vi "UHR-Fleezers Control (host) - 12.1.vi"() -> ()   [LabVIEW 2012] (continued)
          tunnel: "Setpoints (V)" -> [w3405 w3420]
          tunnel: w3394 -> [_ w3414]
          frame False {
            n2043 = Multiply(x=3276.7, y=w3405) -> (x*y=w3406:cluster{"Set 1":dbl, "Set 2":dbl})
            n2044 = To Word Integer(number=w3406) -> (16bit integer=w3404:cluster{"Set 1":i16, "Set 2":i16})
          }
          frame True {
            n2045 = Unbundle By Name(w3414) -> ("Set 1"=w3413:dbl, "Set 2"=w3412:dbl)
            n2046 = Unbundle By Name(w3420) -> ("Set 1"=w3419:dbl, "Set 2"=w3418:dbl)
            n2047 = Unbundle By Name(w3417) -> ("Set 1"=w3416:bool, "Set 2"=w3415:bool)
            n2048 = Select(t=w3413, s=w3416, f=w3419) -> (s? t:f=w3411:dbl)
            n2049 = Select(t=w3412, s=w3415, f=w3418) -> (s? t:f=w3410:dbl)
            n2050 = Bundle By Name(cluster=w3420, "Set 1"=w3411, "Set 2"=w3410) -> (w3408:cluster{"Set 1":dbl, "Set 2":dbl})
            n2051 = local write "Setpoints (V)"(w3408) -> ()
            n2052 = Multiply(x=3276.7, y=w3408) -> (x*y=w3409:cluster{"Set 1":dbl, "Set 2":dbl})
            n2053 = To Word Integer(number=w3409) -> (16bit integer=w3421:cluster{"Set 1":i16, "Set 2":i16})
          }
        }
        n2054 = Unbundle By Name(w3393) -> ("Set 1"=w3392:i16, "Set 2"=w3391:i16)
        n2055 = xnode "Read/Write Control"("FPGA VI Reference In"=w3389, "error in"=w3388, "FB Setpoint Set 1"=w3392, "FB Setpoint Set 2"=w3391) -> ("error out"=w3387:errorcluster)  [unwired: 1 out]
      }
      event "Invert GI": Value Change {
        n2056 = event-data() -> ()  [unwired: 7 out]
        n2057 = xnode "Read/Write Control"("FPGA VI Reference In"=w3426, "error in"=w3424, "Invert GI"="Invert GI", "Invert GI 2"="Invert GI") -> ("error out"=w3425:errorcluster)  [unwired: 1 out]
      }
      event "Green FB Setpoint (mV)", "Green FB Gains", "Green FB On/Off", "Current When FB OFF (%)", "Green int current ON count adj": Value Change {
        n2058 = event-data() -> ()  [unwired: 7 out]
        n2059 = local read "Green FB Setpoint (mV)"() -> (w3437:dbl)
        n2060 = local read "Current When FB OFF (%)"() -> (w3440:dbl)
        n2061 = Multiply(x=w3437, y=3.2767) -> (x*y=w3436:dbl)
        n2062 = Multiply(x=w3440, y=655.35) -> (x*y=w3441:dbl)
        n2063 = To Unsigned Word Integer(number=w3441) -> (unsigned 16bit integer=w3439:u16)
        n2064 = local read "Green int current ON count adj"() -> (w3443:u32)
        n2065 = local read "Green Laser ON/Interlacing"() -> (w3434:bool)
        n2066 = local read "Green FB Gains"() -> (w3430:T9)
        n2067 = local read "Green laser mode"() -> (w3433:enum32{"Laser ON", "Laser OFF", "Interlace"})
        n2068 = local read "Green FB On/Off"() -> (w3444:bool)
        n2069 = Equal?(x=w3433, y=enum32{"Laser ON", "Laser OFF", "Interlace"}."Interlace") -> (x = y?=w3431:bool)
        n2070 = Unbundle By Name(w3430) -> ("proportional gain (Kc)"=w3429:i16, "integral gain (Kc*Ts/Ti)"=w3428:i16, "derivative gain (Kc*Td/Ts)"=w3427:i16)
        n2071 = Compound Arithmetic op=AND(w3431, w3444, w3434) -> (w3435:bool)
        n2072 = xnode "Read/Write Control"("FPGA VI Reference In"=w3447, "error in"=w3446, "Green FB Setpoint"=w3436, "Green FB On/Off"=w3435, "Current Out"=w3439, "Green int current ON count adj"=w3443, "P3"=w3429, "I3"=w3428, "D3"=w3427) -> ("error out"=w3445:errorcluster)  [unwired: 1 out]
      }
      event "Green laser mode", "Green Laser ON/Interlacing": Value Change {
        n2073 = event-data() -> ()  [unwired: 7 out]
        n2074 = local write "Green Laser ON/OFF"("Green Laser ON/Interlacing") -> ()
        n2075 = case shown="True" "Green Laser ON/Interlacing" {
          tunnel: "Green laser mode" -> [_ w3461]
          tunnel: [enum32{"Laser ON", "Laser OFF", "Interlace"}."Laser OFF" ("Green laser mode") w3461] -> w3450
          tunnel: [FALSE w3457] -> w3449
          frame False {
          }
          frame True {
            n2076 = local read "Green FB On/Off"() -> (w3458:bool)
            n2077 = Equal?(x=w3461, y=enum32{"Laser ON", "Laser OFF", "Interlace"}."Interlace") -> (x = y?=w3459:bool)
            n2078 = And(x=w3459, y=w3458) -> (x .and. y?=w3457:bool)
          }
        }
        n2079 = xnode "Read/Write Control"("FPGA VI Reference In"=w3454, "error in"=w3452, "Operating Mode"=w3450, "Operating Mode 2"=w3450, "Green FB On/Off"=w3449) -> ("error out"=w3453:errorcluster)  [unwired: 1 out]
      }
      event "Green Laser ON/OFF": Value Change {
        n2080 = event-data() -> ()  [unwired: 7 out]
        n2081 = property on="Green Laser ON/Interlacing" class="Bool (strict)"("Val(Sgnl)"="Green Laser ON/OFF") -> ()  [unwired: 2 in, 2 out]
      }
      event "Test ttrig": Value Change {
        n2082 = event-data() -> ()  [unwired: 7 out]
        n2083 = xnode "Read/Write Control"("FPGA VI Reference In"=w3466, "error in"=w3465, "TTrig?"=TRUE) -> ("error out"=w3464:errorcluster)  [unwired: 1 out]
      }
      event "Neg. TTrig FPGA": Value Change {
        n2084 = event-data() -> ()  [unwired: 7 out]
        n2085 = xnode "Read/Write Control"("FPGA VI Reference In"=w3470, "error in"=w3469, "TTrig Negate Pos"="Neg. TTrig FPGA") -> ()  [unwired: 2 out]
      }
      event "- phase (APD 1 Gate)", "+ phase (APD 1 Gate)": Value Change {
        n2086 = event-data() -> ()  [unwired: 7 out]
        n2087 = local read "Phase Adj. (APD 1 Gate)"() -> (w3471:i16)
        n2088 = Negate(x=w3471) -> (-x=w3479:i16)
        n2089 = Select(t=w3479, s="- phase (APD 1 Gate)", f=w3471) -> (s? t:f=w3478:i16)
        n2090 = Or(x="- phase (APD 1 Gate)", y="+ phase (APD 1 Gate)") -> (x .or. y?=w3474:bool)
        n2091 = xnode "Read/Write Control"("FPGA VI Reference In"=w3481, "error in"=w3480, "Phase count adjustment (APD 1 Gate)"=w3478) -> ("FPGA VI Reference Out"=w3476:T18, "error out"=w3477:errorcluster)
        n2092 = xnode "Read/Write Control"("FPGA VI Reference In"=w3476, "error in"=w3477, "+ phase (APD 1 Gate)"=w3474) -> ("error out"=w3475:errorcluster)  [unwired: 1 out]
      }
      event "+ phase (APD 2 Gate)", "- phase (APD 2 Gate)": Value Change {
        n2093 = event-data() -> ()  [unwired: 7 out]
        n2094 = local read "Phase Adj. (APD 2 Gate)"() -> (w3482:i16)
        n2095 = Negate(x=w3482) -> (-x=w3490:i16)
        n2096 = Select(t=w3490, s="- phase (APD 2 Gate)", f=w3482) -> (s? t:f=w3489:i16)
        n2097 = Or(x="- phase (APD 2 Gate)", y="+ phase (APD 2 Gate)") -> (x .or. y?=w3485:bool)
        n2098 = xnode "Read/Write Control"("FPGA VI Reference In"=w3492, "error in"=w3491, "Phase count adjustment (APD 2 Gate)"=w3489) -> ("FPGA VI Reference Out"=w3487:T18, "error out"=w3488:errorcluster)
        n2099 = xnode "Read/Write Control"("FPGA VI Reference In"=w3487, "error in"=w3488, "+ phase (APD 2 Gate)"=w3485) -> ("error out"=w3486:errorcluster)  [unwired: 1 out]
      }
      event "Phase Adj. (APD Acq)", "+ phase (APD Acq)", "- phase (APD Acq)": Value Change {
        n2100 = event-data() -> ()  [unwired: 7 out]
        n2101 = local read "Phase Adj. (APD Acq)"() -> (w3495:i16)
        n2102 = Negate(x=w3495) -> (-x=w3501:i16)
        n2103 = Select(t=w3501, s="+ phase (APD Acq)", f=w3495) -> (s? t:f=w3500:i16)
        n2104 = Or(x="+ phase (APD Acq)", y="- phase (APD Acq)") -> (x .or. y?=w3496:bool)
        n2105 = xnode "Read/Write Control"("FPGA VI Reference In"=w3503, "error in"=w3502, "Phase Count Adjustment (APD Acq)"=w3500) -> ("FPGA VI Reference Out"=w3498:T18, "error out"=w3499:errorcluster)
        n2106 = xnode "Read/Write Control"("FPGA VI Reference In"=w3498, "error in"=w3499, "+ phase (APD Acq)"=w3496) -> ("error out"=w3497:errorcluster)  [unwired: 1 out]
      }
      event "Phase adj. (GI)", "+ phase (GI)", "- phase (GI)": Value Change {
        n2107 = event-data() -> ()  [unwired: 7 out]
        n2108 = Negate(x="Phase adj. (GI)") -> (-x=w3512:i16)
        n2109 = Select(t=w3512, s="+ phase (GI)", f="Phase adj. (GI)") -> (s? t:f=w3511:i16)
        n2110 = Or(x="+ phase (GI)", y="- phase (GI)") -> (x .or. y?=w3507:bool)
        n2111 = xnode "Read/Write Control"("FPGA VI Reference In"=w3514, "error in"=w3513, "Phase count adjustment (GI)"=w3511) -> ("FPGA VI Reference Out"=w3509:T18, "error out"=w3510:errorcluster)
        n2112 = xnode "Read/Write Control"("FPGA VI Reference In"=w3509, "error in"=w3510, "+ phase (GI)"=w3507) -> ("error out"=w3508:errorcluster)  [unwired: 1 out]
      }
      event "Phase adj. (GI) 2", "+ phase (GI) 2", "- phase (GI) 2": Value Change {
        n2113 = event-data() -> ()  [unwired: 7 out]
        n2114 = Negate(x="Phase adj. (GI) 2") -> (-x=w3523:i16)
        n2115 = Select(t=w3523, s="+ phase (GI) 2", f="Phase adj. (GI) 2") -> (s? t:f=w3522:i16)
        n2116 = Or(x="+ phase (GI) 2", y="- phase (GI) 2") -> (x .or. y?=w3518:bool)
        n2117 = xnode "Read/Write Control"("FPGA VI Reference In"=w3525, "error in"=w3524, "Phase count adjustment (GI) 2"=w3522) -> ("FPGA VI Reference Out"=w3520:T18, "error out"=w3521:errorcluster)
        n2118 = xnode "Read/Write Control"("FPGA VI Reference In"=w3520, "error in"=w3521, "+ phase (GI) 2"=w3518) -> ("error out"=w3519:errorcluster)  [unwired: 1 out]
      }
      event "Phase adj. (Green FB)", "- phase (Green FB)", "+ phase (Green FB)": Value Change {
        n2119 = event-data() -> ()  [unwired: 7 out]
        n2120 = Negate(x="Phase adj. (Green FB)") -> (-x=w3534:i16)
        n2121 = Select(t=w3534, s="+ phase (Green FB)", f="Phase adj. (Green FB)") -> (s? t:f=w3533:i16)
        n2122 = Or(x="+ phase (Green FB)", y="- phase (Green FB)") -> (x .or. y?=w3529:bool)
        n2123 = xnode "Read/Write Control"("FPGA VI Reference In"=w3536, "error in"=w3535, "Phase count adjustment (Green FB)"=w3533) -> ("FPGA VI Reference Out"=w3531:T18, "error out"=w3532:errorcluster)
        n2124 = xnode "Read/Write Control"("FPGA VI Reference In"=w3531, "error in"=w3532, "+ phase (Green FB)"=w3529) -> ("error out"=w3530:errorcluster)  [unwired: 1 out]
      }
      event "Invert APD Gate", "APD Gate ON Count", "APD Gate OFF Count", "APD Gate", "APD Integration Time (s)", "APD 1 AO Mult.", "APD 2 AO Mult.", "On one out of X cycles": Value Change {
        n2125 = event-data() -> ()  [unwired: 7 out]
        n2126 = Add(x="GI Frequency, ON count", y="GI Frequency, OFF count") -> (x+y=w3540:u32)
        n2127 = Add(x="APD Gate ON Count", y="APD Gate OFF Count") -> (x+y=w3553:u32)
        n2128 = Multiply(x="On one out of X cycles", y=w3540) -> (x*y=w3537:u32)
        "Green FB Count" <- w3537
        n2129 = Subtract(x=w3537, y="GI Frequency, ON count") -> (x-y=w3538:u32)
        n2130 = Multiply(x=w3553, y="On one out of X cycles") -> (x*y=w3552:u32)
        n2131 = Subtract(x=w3552, y="APD Gate ON Count") -> (x-y=w3551:u32)
        n2132 = local read "DMA Update Period (s)"() -> (w3554:dbl)
        n2133 = Multiply(x="APD Integration Time (s)", y=40000000.0) -> (x*y=w3559:dbl)
        n2134 = Reciprocal(x="APD Integration Time (s)") -> (1/x=→"APD Acq Rate (Hz)":dbl)
        n2135 = To Unsigned Long Integer(number=w3559) -> (unsigned 32bit integer=w3543:u32)
        "APD Int. Count" <- w3543
        n2136 = xnode "Read/Write Control"("FPGA VI Reference In"=w3563, "error in"=w3562, "Invert APD Gate"="Invert APD Gate", "APD Gate ON Count"="APD Gate ON Count", "APD Gate OFF Count"=w3551, "APD Acq Rate Count"=w3543, "APD Gate Operating Mode"="APD Gate", "APD 1 AO scale factor"="APD 1 AO Mult.", "APD 2 AO scale factor"="APD 2 AO Mult.", "Green interlace ON count"="GI Frequency, ON count", "Green interlace OFF count"=w3538, "Green interlace ON count 2"="GI Frequency, ON count", "Green interlace OFF count 2"=w3538, "Green FB Count"=w3537) -> ("error out"=w3561:errorcluster)  [unwired: 1 out]
        n2137 = Divide(x=w3554, y="APD Integration Time (s)") -> (x/y=w3557:dbl)
        n2138 = Multiply(x=2.0, y=w3557) -> (x*y=w3556:dbl)
        n2139 = local write "APD Samples/FIFO Acq."(w3557) -> ()
        n2140 = local write "APD Elements/DMA read"(w3556) -> ()
      }
      event "Number of F/B Scans (AOD)", "Scan Speed (nm/s)", "Scan BD", "Initial delta (MHz)", "Step Size (nm)", "Scan Range (nm)": Value Change {
        w3625 = 123.0  # AOM cal (nm/MHz)
        n2141 = event-data() -> ()  [unwired: 7 out]
        n2142 = local read "BD 1 Frequency 1 (MHz)"() -> (w3608:dbl)
        n2143 = local read "AOM X Cal (nm/MHz)"() -> (w3600:dbl)
        n2144 = local read "X RF Frequency Limits (MHz)"() -> (w3612:T15)
        n2145 = local read "Y RF Frequency Limits (MHz)"() -> (w3609:T15)
        n2146 = local read "BD 2 Frequency 1 (MHz)"() -> (w3614:dbl)
        n2147 = Negate(x="Scan Range (nm)") -> (-x=w3578:dbl)
        n2148 = Divide(x=w3578, y=w3600) -> (x/y=w3582:dbl)
        n2149 = Select(t=w3612, s="Scan BD", f=w3609) -> (s? t:f=w3611:T15)
        n2150 = Select(t=w3608, s="Scan BD", f=w3614) -> (s? t:f=w3613:dbl)
        n2151 = Unbundle By Name(w3611) -> ("Maximum"=w3620:dbl, "Minimum"=w3619:dbl)
        n2152 = Add(x=w3582, y=w3613) -> (x+y=w3617:dbl)
        n2153 = Divide(x=w3578, y="Step Size (nm)") -> (x/y=w3597:dbl)
        n2154 = Divide(x="Step Size (nm)", y=w3600) -> (x/y=w3606:dbl)
        n2155 = Absolute Value(x=w3597) -> (abs(x)=w3581:dbl)
        n2156 = Sign(1:w3578) -> (0:w3579:dbl)
        n2157 = In Range and Coerce(upper limit=w3620, x=w3617, lower limit=w3619) -> (coerced(x)=w3616:dbl, In Range?=w3618:bool)
        n2158 = To Unsigned Quad Integer(1:w3581) -> (0:w3596:u64)
        "Scan steps (AOD)" <- w3596
        n2159 = call "IR AOM freq to word.vi"("Frequency In (MHz)"=w3606) -> ("Frequency Word Out (double)"=w3603:dbl)
        n2160 = Multiply(x=w3579, y=w3603) -> (x*y=w3580:dbl)
        n2161 = Subtract(x=w3617, y=w3616) -> (x-y=w3615:dbl)
        n2162 = To Quad Integer(1:w3580) -> (0:w3602:i64)
        "Incr. int (AOD)" <- w3602
        n2163 = Subtract(x=w3582, y=w3615) -> (x-y=w3601:dbl)
        "Scan Range (MHz)" <- w3601
        n2164 = Select(t=w3582, s=w3618, f=w3601) -> (s? t:f=w3621:dbl)
        n2165 = Multiply(x=w3601, y=w3600) -> (x*y=w3599:dbl)
        n2166 = Decrement(x=w3596) -> (x-1=w3649:u64)
        n2167 = Negate(x=w3599) -> (-x=w3595:dbl)
        n2168 = local write "Scan Range (nm)"(w3595) -> ()
        n2169 = Divide(x=w3621, y=w3649) -> (x/y=w3605:dbl)
        "Scan Increment (MHz)" <- w3605
        n2170 = call "IR AOM freq to word.vi"("Frequency In (MHz)"=w3605) -> ("Frequency Word Out (double)"=w3604:dbl)
        n2171 = Divide(x="Step Size (nm)", y="Scan Speed (nm/s)") -> (x/y=w3592:dbl)
        n2172 = To Quad Integer(1:w3604) -> ()  [unwired: 1 out]
        n2173 = local read "Number Interlace Sets"() -> (w3576:u8)
        n2174 = local read "AI Count (ticks)"() -> (w3577:u32)
        n2175 = local read "Total Counts (ticks)"() -> (w3575:u32)
        n2176 = local read "# Samples/trap"() -> (w3607:u32)
        n2177 = Multiply(x=w3577, y=w3576) -> (x*y=w3574:u32)
        n2178 = Divide(x=w3575, y=w3574) -> (x/y=w3573:dbl)
        n2179 = Select(t=w3608, s="Scan BD", f=w3614) -> (s? t:f=w3646:dbl)
        "Initial freq. (MHz)" <- w3646
        n2180 = Add(x=w3621, y=w3646) -> (x+y=→"Final freq. (MHz)":dbl)
        n2181 = Divide(x=w3575, y=40000000.0) -> (x/y=w3591:dbl)
        n2182 = Divide(x=w3592, y=w3591) -> (x/y=w3590:dbl)
        n2183 = To Unsigned Quad Integer(1:w3590) -> (0:w3565:u64)
        n2184 = Quotient & Remainder(x=w3565, y=u64 2) -> (x-y*floor(x/y)=w3569:u64)  [unwired: 1 out]
        n2185 = Equal?(x=w3569, y=u64 0) -> (x = y?=w3567:bool)
        n2186 = Decrement(x=w3565) -> (x-1=w3566:u64)
        n2187 = Select(t=w3565, s=w3567, f=w3566) -> (s? t:f=w3564:u64)
        "Cycles/step (AOD)" <- w3564
        n2188 = xnode "Read/Write Control"("FPGA VI Reference In"=w3657, "error in"=w3656, "Scan steps"=w3596, "Number of scans"="Number of F/B Scans (AOD)", "Cycles per step"=w3564, "Scan freq.  increment"=w3602, "Scan BD"="Scan BD") -> ("error out"=w3655:errorcluster)  [unwired: 1 out]
        n2189 = Multiply(x=w3596, y=w3564) -> (x*y=w3650:u64)
        n2190 = Multiply(x=w3650, y=u64 2) -> (x*y=w3572:u64)
        n2191 = Multiply(x=w3573, y=w3572) -> (x*y=w3571:dbl)
        "Data points/scan (f/b)" <- w3571
        n2192 = Multiply(x=w3571, y="Number of F/B Scans (AOD)") -> (x*y=w3653:dbl)
        "Data points/scans" <- w3653
        n2193 = Divide(x=w3653, y=w3607) -> (x/y=→"N sets should be saved":dbl)
        n2194 = Multiply(x=w3650, y=w3591) -> (x*y=w3589:dbl)
        "Time/Scan (s) (AOD)" <- w3589
        n2195 = Select(t=w3621, s="Scan BD", f=0.0) -> (s? t:f=w3647:dbl)
        n2196 = Select(t=0.0, s="Scan BD", f=w3621) -> (s? t:f=w3643:dbl)
        n2197 = local read "BD 2 Frequency 2 (MHz)"() -> (w3639:dbl)
        n2198 = local read "BD 1 Frequency 2 (MHz)"() -> (w3642:dbl)
        n2199 = Add(x=w3643, y=w3614) -> (x+y=w3640:dbl)
        n2200 = Add(x=w3608, y=w3647) -> (x+y=w3641:dbl)
        n2201 = Multiply(x=w3589, y=2.0) -> (x*y=w3588:dbl)
        n2202 = Multiply(x=w3588, y="Number of F/B Scans (AOD)") -> (x*y=w3585:dbl)
        n2203 = Divide(x=w3585, y=60.0) -> (x/y=→"Time to Finish All (min)":dbl)
        n2204 = Add(x="Trap 2 Bead Size (nm)", y="Trap 1 Bead Size (nm)") -> (x+y=w3629:dbl)
        n2205 = Divide(x=w3629, y=2.0) -> (x/y=w3623:dbl)
        n2206 = local read "Initial delta (MHz)"() -> (w3626:dbl)
        n2207 = Subtract(x=w3640, y=w3639) -> (x-y=w3637:dbl)
        n2208 = Subtract(x=w3641, y=w3642) -> (x-y=w3638:dbl)
        n2209 = Square(x=w3637) -> (x^2=w3636:dbl)
        n2210 = Square(x=w3638) -> (x^2=w3635:dbl)
        n2211 = Add(x=w3635, y=w3636) -> (x+y=w3634:dbl)
        n2212 = Square Root(x=w3634) -> (sqrt(x)=w3633:dbl)
        "Final delta (MHz)" <- w3633
        n2213 = Multiply(x=w3625, y=w3633) -> (x*y=w3632:dbl)
        n2214 = Multiply(x=w3626, y=w3625) -> (x*y=w3624:dbl)
        n2215 = Subtract(x=w3624, y=w3623) -> (x-y=→"Initial sep (nm)":dbl)
        n2216 = Subtract(x=w3632, y=w3623) -> (x-y=→"Final sep (nm)":dbl)
      }
      event "Freq or Amp switch first", "Swap F1 and F2", "Freq switch delay", "Amp switch delay": Value Change {
        n2217 = event-data() -> ()  [unwired: 7 out]
        n2218 = local read "Amp switch delay"() -> (w3658:u16)
        n2219 = local read "Swap F1 and F2"() -> (w3659:bool)
        n2220 = xnode "Read/Write Control"("FPGA VI Reference In"=w3662, "error in"=w3661, "Swap F1 and F2"=w3659, "Amp switch delay"=w3658) -> ("error out"=w3660:errorcluster)  [unwired: 1 out]
      }
      event "Scan steps (MCL)", "Number of scans (MCL)", "Scan Range (V)\n(of steps)", "2D or 1D Scan", "N APD Samp/step", "Fast Scan Dir", "Continuous MCL Scanning", "Scan lines (y)": Value Change {
        w3664 = 32767.0 ("y")
        n2221 = event-data() -> ()  [unwired: 7 out]
        n2222 = Select(t="Scan lines (y)", s="2D or 1D Scan", f="Number of scans (MCL)") -> (s? t:f=w3669:u64)
        n2223 = Decrement(x="Scan steps (MCL)") -> (x-1=w3685:u64)
        n2224 = Divide(x="Scan Range (V)\n(of steps)", y=w3685) -> (x/y=w3684:dbl)
        "Desired Scan Incr (V)" <- w3684
        n2225 = local read "APD Integration Time (s)"() -> (w3677:dbl)
        n2226 = Multiply(x=w3684, y=w3664) -> (x*y=w3693:dbl)
        n2227 = Divide(x=w3693, y=10.0) -> (x/y=w3683:dbl)
        "Desired incr (int)" <- w3683
        n2228 = local read "Update Count (MCL)"() -> (w3689:u32)
        n2229 = Round Toward -Infinity(1:w3683) -> (0:w3692:dbl)
        n2230 = To Word Integer(number=w3692) -> (16bit integer=w3667:i16)
        "Actual Incr. int (MCL)" <- w3667
        n2231 = Multiply(x=w3677, y=40000000.0) -> (x*y=w3690:dbl)
        n2232 = Divide(x=w3690, y=w3689) -> (x/y=w3688:dbl)
        n2233 = Multiply(x=i16 10, y=w3667) -> (x*y=w3665:i16)
        n2234 = Multiply(x="N APD Samp/step", y=w3688) -> (x*y=w3687:dbl)
        "Cycles/step (MCL)" <- w3687
        n2235 = Divide(x=w3665, y=w3664) -> (x/y=→"Actual MCL Inc (V)":dbl)
        n2236 = Multiply(x="N APD Samp/step", y="Scan steps (MCL)") -> (x*y=w3679:dbl)
        n2237 = local read "APD Samples/FIFO Acq."() -> (w3676:dbl)
        n2238 = Multiply(x=w3679, y=u64 2) -> (x*y=w3678:dbl)
        "Data points/scan (f+b)" <- w3678
        n2239 = Multiply(x=w3678, y=w3669) -> (x*y=w3696:dbl)
        "Data points/scans (MCL)" <- w3696
        n2240 = Multiply(x=w3677, y=w3678) -> (x*y=w3670:dbl)
        "Time/f+b scan (s) (MCL)" <- w3670
        n2241 = Divide(x=w3696, y=w3676) -> (x/y=→"N sets should be saved (MCL)":dbl)
        n2242 = Multiply(x=w3670, y=w3669) -> (x*y=→"Total Time (s)":dbl)
        n2243 = Not(x="Fast Scan Dir") -> (.not. x?=w3674:bool)
        n2244 = xnode "Read/Write Control"("FPGA VI Reference In"=w3700, "error in"=w3699, "Scan steps (MCL)"="Scan steps (MCL)", "Number of scans (MCL)"=w3669, "Cycles per step (MCL)"=w3687, "Scan freq.  increment (MCL)"=w3667, "1D or 2D Scan?"="2D or 1D Scan", "MCL Scan Axis"=w3674, "Cont. Scan (MCL)"="Continuous MCL Scanning") -> ("error out"=w3698:errorcluster)  [unwired: 1 out]
      }
      event "Read Cal": Value Change {
        w3702 = 1000.0 ("y")
        n2245 = event-data() -> ()  [unwired: 7 out]
        n2246 = local read "Save file name"() -> (w3727:path)
        n2247 = local write "Read Cal"(FALSE ("Read Cal")) -> ()
        n2248 = Strip Path(path=w3727) -> (stripped path=w3726:path)  [unwired: 1 out]
        n2249 = Path To String(path=w3726) -> (string=w3725:string)
        n2250 = Concatenate Strings(w3725, "\\current.cal" ("string")) -> (w3723:string)
        n2251 = String To Path(string=w3723) -> (path=w3722:path)
        n2252 = Open/Create/Replace File(file path (use dialog)=w3722, operation (0:open)=T34."open", access (0:read/write)=enum16{"read/write", "read-only", "write-only"}."read-only") -> (refnum out=w3730:refnum<file>, error out=w3716:errorcluster)  [unwired: 1 in, 3 out]
        n2253 = Deny Access(4:w3716, 7:w3730) -> (0:w3715:errorcluster, 3:w3721:refnum<file>)  [unwired: 1 out]
        n2254 = Read from Binary File(5:0.0, 8:w3715, 9:T35."big-endian, network order" ("byte order (0:big-endian, network order)"), 10:-1 ("count (1)"), 11:w3721) -> (0:w3714:errorcluster, 2:w3712:dbl[], 3:w3717:refnum<file>)  [unwired: 2 out]
        n2255 = Array To Cluster(array=w3712) -> (cluster=w3711:T43)
        n2256 = Unbundle(w3711) -> ("[0]"=w3710:dbl, "[1]"=w3709:dbl, "[2]"=w3708:dbl, "[3]"=w3707:dbl, "[4]"=w3706:dbl, "[5]"=w3705:dbl)
        n2257 = Close File(refnum=w3717, error in=w3714) -> (error out=→"Read cal error":errorcluster)  [unwired: 1 out]
        n2258 = Multiply(x=w3705, y=w3702) -> (x*y=w3703:dbl)
        n2259 = local write "T2 kappa_x (pN/nm)"(w3707) -> ()
        n2260 = local write "T1 kappa_x (pN/nm)"(w3708) -> ()
        n2261 = local write "T1 alpha_x (nm/V)"(w3710) -> ()
        n2262 = local write "T2 alpha_x (nm/V)"(w3709) -> ()
        n2263 = Multiply(x=w3706, y=w3702) -> (x*y=w3704:dbl)
        n2264 = local write "T1 offset_x (mV)"(w3704) -> ()
        n2265 = local write "T2 offset_x (mV)"(w3703) -> ()
      }
      event "Abort MCL Scan": Value Change {
        n2266 = event-data() -> ()  [unwired: 7 out]
        n2267 = local write "MCL Scanning"(FALSE ("MCL Scanning")) -> ()
        n2268 = xnode "Read/Write Control"("FPGA VI Reference In"=w3735, "error in"=w3734, "Abort scan (MCL)"="Abort MCL Scan") -> ("error out"=w3733:errorcluster)  [unwired: 1 out]
      }
      event "Update Count (MCL)": Value Change {
        n2269 = event-data() -> ()  [unwired: 7 out]
        n2270 = xnode "Read/Write Control"("FPGA VI Reference In"=w3739, "error in"=w3738, "MCL count"="Update Count (MCL)") -> ("error out"=w3737:errorcluster)  [unwired: 1 out]
      }
      event "Phase adjust (MCL)", "+ phase (MCL)", "- phase (MCL)": Value Change {
        n2271 = event-data() -> ()  [unwired: 7 out]
        n2272 = Negate(x="Phase adjust (MCL)") -> (-x=w3748:i16)
        n2273 = Select(t=w3748, s="- phase (MCL)", f="Phase adjust (MCL)") -> (s? t:f=w3746:i16)
        n2274 = Or(x="- phase (MCL)", y="+ phase (MCL)") -> (x .or. y?=w3741:bool)
        n2275 = xnode "Read/Write Control"("FPGA VI Reference In"=w3750, "error in"=w3749, "Phase count adjustment (MCL)"=w3746) -> ("FPGA VI Reference Out"=w3742:T18, "error out"=w3743:errorcluster)
        n2276 = xnode "Read/Write Control"("FPGA VI Reference In"=w3742, "error in"=w3743, "+ phase (MCL)"=w3741) -> ("error out"=w3740:errorcluster)  [unwired: 1 out]
      }
      event "Abort AOD Scan": Value Change {
        n2277 = event-data() -> ()  [unwired: 7 out]
        n2278 = xnode "Read/Write Control"("FPGA VI Reference In"=w3754, "error in"=w3753, "Abort scan"="Abort AOD Scan") -> ("error out"=w3752:errorcluster)  [unwired: 1 out]
      }
      event "Continuous AOD Scanning": Value Change {
        n2279 = event-data() -> ()  [unwired: 7 out]
        n2280 = xnode "Read/Write Control"("FPGA VI Reference In"=w3758, "error in"=w3757, "Cont. Scan"="Continuous AOD Scanning") -> ("error out"=w3756:errorcluster)  [unwired: 1 out]
      }
      event "Index": Value Change {
        n2281 = event-data() -> ()  [unwired: 7 out]
        n2282 = call "Create new save file.vi"("Insert"="", "Ext"=".dat" ("string"), "Index In"="Index") -> ("Path Out"=→"Save file name":path, "Index Out"=w3759:dbl)
        "Save index" <- w3759
        n2283 = local write "Index"(w3759) -> ()
      }
      event "AO1", "AO2": Value Change {
        w3774 = 10.0 ("y")
        w3773 = 32767.0 ("y")
        n2284 = event-data() -> ()  [unwired: 7 out]
        n2285 = local read "AO2"() -> (w3772:dbl)
        n2286 = local read "AO1"() -> (w3769:dbl)
        n2287 = Multiply(x=w3769, y=w3773) -> (x*y=w3768:dbl)
        n2288 = Multiply(x=w3772, y=w3773) -> (x*y=w3771:dbl)
        n2289 = Divide(x=w3768, y=w3774) -> (x/y=w3767:dbl)
        n2290 = Divide(x=w3771, y=w3774) -> (x/y=w3770:dbl)
        n2291 = To Word Integer(number=w3767) -> (16bit integer=w3775:i16)
        n2292 = To Word Integer(number=w3770) -> (16bit integer=w3776:i16)
        n2293 = xnode "Read/Write Control"("FPGA VI Reference In"=w3766, "error in"=w3765, "AO1"=w3775, "AO2"=w3776) -> ("error out"=w3764:errorcluster)  [unwired: 1 out]
      }
      event "Inject Pump 1": Value Change {
        n2294 = event-data() -> ()  [unwired: 7 out]
        n2295 = local read "Use Harvard pumps\nfor beads (else Chemyx)"() -> (w3778:bool)
        n2296 = case shown="True" w3778 {
          tunnel: "Inject Pump 1" -> [w3782 w3820]
          tunnel: w3777 -> [_ w3821]
          frame False {
            n2297 = local read "Pump write delay (ms)"() -> (w3781:dbl)
            n2298 = local read "Chemyx Syringe Pump Serial Port"() -> (w3780:refnum<visa-resource-name>)
            n2299 = case shown="True" w3782 {
              tunnel: w3781 -> [w3788 w3802]
              tunnel: w3780 -> [w3785 w3801]
              frame False {
                n2300 = flat-sequence {
                  tunnel: w3785 -> [w3789]
                  tunnel: [w3789] -> w3786
                  tunnel: w3788 -> [_]
                  tunnel: [w3792] -> w3787
                  tunnel: w3786 -> [w3792]
                  tunnel: w3787 -> [w3793]
                  tunnel: [w3793] -> w3783
                  tunnel: [w3795] -> w3784
                  tunnel: w3783 -> [w3795]
                  tunnel: w3784 -> [w3797]
                  frame #0 {
                    n2301 = call "Write to pump.vi"("string"="enter pump1", "VISA resource name"=w3789) -> ()  [unwired: 1 out]
                  }
                  frame #1 {
                    n2302 = Wait (ms)(milliseconds to wait="Pump pause delay (ms)") -> ()  [unwired: 1 out]
                  }
                  frame #2 {
                    n2303 = call "Write to pump.vi"("string"="stop", "VISA resource name"=w3793) -> ()  [unwired: 1 out]
                  }
                  frame #3 {
                    n2304 = Wait (ms)(milliseconds to wait=u32 500) -> ()  [unwired: 1 out]
                  }
                  frame #4 {
                    n2305 = call "Write to pump.vi"("string"="stop", "VISA resource name"=w3797) -> ()  [unwired: 1 out]
                  }
                }
              }
              frame True {
                n2306 = flat-sequence {
                  tunnel: w3801 -> [w3811]
                  tunnel: w3802 -> [w3806]
                  tunnel: w3802 -> [w3813]
                  tunnel: w3801 -> [w3814]
                  tunnel: [w3814] -> w3799
                  tunnel: [w3816] -> w3800
                  tunnel: w3799 -> [w3816]
                  tunnel: w3800 -> [w3818]
                  frame #0 {
                    n2307 = local read "All Pump Parameters"() -> (w3805:T5)
                    n2308 = Unbundle By Name(w3805) -> ("Pump 1"=w3812:T44)
                    n2309 = call "Set pump parameters.vi"("Pump write delay (ms)"=w3806, "Volume (uL)"="Ch 1 Inject Volume (uL)", "Rate (uL/h)"="Ch 1 Inject Rate (ul/h)", "Units"=4.0, "Pump #"=1.0, "Pump Parameters In"=w3812, "VISA resource name"=w3811) -> ("Pump Parameters Out"=w3804:T44)  [unwired: 3 in]
                    n2310 = Bundle By Name(cluster=w3805, "Pump 1"=w3804) -> (w3803:T5)
                    n2311 = local write "All Pump Parameters"(w3803) -> ()
                  }
                  frame #1 {
                    n2312 = Wait (ms)(milliseconds to wait=w3813) -> ()  [unwired: 1 out]
                  }
                  frame #2 {
                    n2313 = call "Write to pump.vi"("string"="start", "VISA resource name"=w3814) -> ()  [unwired: 1 out]
                  }
                  frame #3 {
                    n2314 = Wait (ms)(milliseconds to wait=u32 500) -> ()  [unwired: 1 out]
                  }
                  frame #4 {
                    n2315 = call "Write to pump.vi"("string"="start", "VISA resource name"=w3818) -> ()  [unwired: 1 out]
                  }
                }
              }
            }
          }
          frame True {
            n2316 = case shown="False" w3820 {
              tunnel: w3821 -> [w3822 w3832]
              frame False {
                n2317 = flat-sequence {
                  tunnel: w3822 -> [w3824]
                  frame #0 {
                    n2318 = local write "Flushing P1"(FALSE ("Flushing P1")) -> ()
                    n2319 = Concatenate Strings("stop" ("string"), "\r") -> (w3826:string)
                    n2320 = VISA Write(VISA resource name=w3824, write buffer=w3826) -> ()  [unwired: 1 in, 3 out]
                  }
                  frame #1 {
                    n2321 = property on="Clear Volume P1" class="Bool (strict)"("Val(Sgnl)"=TRUE ("Value (Signaling)")) -> ()  [unwired: 2 in, 2 out]
                  }
                }
              }
              frame True {
                n2322 = local read "Normal Flow Rate (ul/h) P1"() -> (w3830:dbl)
                n2323 = Number To Decimal String(number=w3830) -> (decimal integer string=w3836:string)  [unwired: 1 in]
                n2324 = Concatenate Strings("irate  " ("string"), w3836, " u/h" ("string"), "\r") -> (w3834:string)
                n2325 = VISA Write(VISA resource name=w3832, write buffer=w3834) -> (VISA resource name out=w3831:refnum<visa-resource-name>)  [unwired: 1 in, 2 out]
                n2326 = Concatenate Strings("irun" ("string"), "\r") -> (w3838:string)
                n2327 = VISA Write(VISA resource name=w3831, write buffer=w3838) -> ()  [unwired: 1 in, 3 out]
              }
            }
          }
        }
      }
      event "Inject Pump 3": Value Change {
        n2328 = event-data() -> ()  [unwired: 7 out]
        n2329 = local read "Use Harvard pumps\nfor beads (else Chemyx)"() -> (w3841:bool)
        n2330 = case shown="True" w3841 {
          tunnel: "Inject Pump 3" -> [w3845 w3884]
          tunnel: w3840 -> [_ w3883]
          frame False {
            n2331 = local read "Pump write delay (ms)"() -> (w3844:dbl)
            n2332 = case shown="True" w3845 {
              tunnel: w3844 -> [w3851 w3865]
              tunnel: "Chemyx Syringe Pump Serial Port" -> [w3848 w3864]
              frame False {
                n2333 = flat-sequence {
                  tunnel: w3848 -> [w3852]
                  tunnel: [w3852] -> w3849
                  tunnel: w3851 -> [_]
                  tunnel: [w3855] -> w3850
                  tunnel: w3849 -> [w3855]
                  tunnel: w3850 -> [w3856]
                  tunnel: [w3856] -> w3846
                  tunnel: [w3858] -> w3847
                  tunnel: w3846 -> [w3858]
                  tunnel: w3847 -> [w3860]
                  frame #0 {
                    n2334 = call "Write to pump.vi"("string"="enter pump3", "VISA resource name"=w3852) -> ()  [unwired: 1 out]
                  }
                  frame #1 {
                    n2335 = local read "Pump pause delay (ms)"() -> (w3854:u32)
                    n2336 = Wait (ms)(milliseconds to wait=w3854) -> ()  [unwired: 1 out]
                  }
                  frame #2 {
                    n2337 = call "Write to pump.vi"("string"="stop", "VISA resource name"=w3856) -> ()  [unwired: 1 out]
                  }
                  frame #3 {
                    n2338 = Wait (ms)(milliseconds to wait=u32 0) -> ()  [unwired: 1 out]
                  }
                  frame #4 {
                    n2339 = call "Write to pump.vi"("string"="stop", "VISA resource name"=w3860) -> ()  [unwired: 1 out]
                  }
                }
              }
              frame True {
                n2340 = flat-sequence {
                  tunnel: w3864 -> [w3874]
                  tunnel: w3865 -> [w3869]
                  tunnel: w3865 -> [w3876]
                  tunnel: w3864 -> [w3877]
                  tunnel: [w3877] -> w3863
                  tunnel: [w3880] -> w3862
                  tunnel: w3863 -> [w3880]
                  tunnel: w3862 -> [w3881]
                  frame #0 {
                    n2341 = local read "All Pump Parameters"() -> (w3868:T5)
                    n2342 = Unbundle By Name(w3868) -> ("Pump 3"=w3875:T44)
                    n2343 = call "Set pump parameters.vi"("Pump write delay (ms)"=w3869, "Volume (uL)"="Ch 3 Inject Volume (uL)", "Rate (uL/h)"="Ch 3 Inject Rate (ul/h)", "Units"=4.0, "Pump #"=3.0, "Pump Parameters In"=w3875, "VISA resource name"=w3874) -> ("Pump Parameters Out"=w3867:T44)  [unwired: 3 in]
                    n2344 = Bundle By Name(cluster=w3868, "Pump 3"=w3867) -> (w3866:T5)
                    n2345 = local write "All Pump Parameters"(w3866) -> ()
                  }
                  frame #1 {
                    n2346 = Wait (ms)(milliseconds to wait=w3876) -> ()  [unwired: 1 out]
                  }
                  frame #2 {
                    n2347 = call "Write to pump.vi"("string"="start", "VISA resource name"=w3877) -> ()  [unwired: 1 out]
                  }
                  frame #3 {
                    n2348 = Wait (ms)(milliseconds to wait=u32 500) -> ()  [unwired: 1 out]
                  }
                  frame #4 {
                    n2349 = call "Write to pump.vi"("string"="start", "VISA resource name"=w3881) -> ()  [unwired: 1 out]
                  }
                }
              }
            }
          }
          frame True {
            n2350 = case shown="False" w3884 {
              tunnel: w3883 -> [w3885 w3892]
              frame False {
                n2351 = flat-sequence {
                  tunnel: w3885 -> [w3887]
                  frame #0 {
                    n2352 = local write "Flushing P3"(FALSE ("Flushing P3")) -> ()
                    n2353 = Concatenate Strings("stop" ("string"), "\r") -> (w3889:string)
                    n2354 = VISA Write(VISA resource name=w3887, write buffer=w3889) -> ()  [unwired: 1 in, 3 out]
                  }
                  frame #1 {
                    n2355 = property on="Clear Volume P3" class="Bool (strict)"("Val(Sgnl)"=TRUE ("Value (Signaling)")) -> ()  [unwired: 2 in, 2 out]
                  }
                }
              }
              frame True {
                n2356 = local read "Normal Flow Rate (ul/h) P3"() -> (w3893:dbl)
                n2357 = Number To Decimal String(number=w3893) -> (decimal integer string=w3899:string)  [unwired: 1 in]
                n2358 = Concatenate Strings("irate  " ("string"), w3899, " u/h" ("string"), "\r") -> (w3897:string)
                n2359 = VISA Write(VISA resource name=w3892, write buffer=w3897) -> (VISA resource name out=w3895:refnum<visa-resource-name>)  [unwired: 1 in, 2 out]
                n2360 = Concatenate Strings("irun" ("string"), "\r") -> (w3901:string)
                n2361 = VISA Write(VISA resource name=w3895, write buffer=w3901) -> ()  [unwired: 1 in, 3 out]
              }
            }
          }
        }
      }
      event "Inject Pump 2": Value Change {
        n2362 = event-data() -> ()  [unwired: 7 out]
        n2363 = local read "Pump write delay (ms)"() -> (w3905:dbl)
        n2364 = flat-sequence {
          tunnel: w3903 -> [w3918]
          tunnel: w3905 -> [w3914]
          tunnel: "Inject Pump 2" -> [_]
          tunnel: w3905 -> [w3920]
          tunnel: w3903 -> [w3921]
          frame #0 {
            n2365 = local read "All Pump Parameters"() -> (w3913:T5)
            n2366 = Multiply(x=60.0, y="Flush Center Ch Rate (ul/m)") -> (x*y=w3910:dbl)
            n2367 = Unbundle By Name(w3913) -> ("Pump 2"=w3919:T44)
            n2368 = call "Set pump parameters.vi"("Pump write delay (ms)"=w3914, "Volume (uL)"="Flush Center Ch Volume (uL)", "Rate (uL/h)"=w3910, "Units"=3.0, "Pump #"=2.0, "Pump Parameters In"=w3919, "VISA resource name"=w3918) -> ("Pump Parameters Out"=w3912:T44)  [unwired: 3 in]
            n2369 = Bundle By Name(cluster=w3913, "Pump 2"=w3912) -> (w3911:T5)
            n2370 = local write "All Pump Parameters"(w3911) -> ()
            n2371 = Add(x="Flush Center Ch Volume (uL)", y="Total Volume\nFlushed (uL)") -> (x+y=w3907:dbl)
            n2372 = local write "Total Volume\nFlushed (uL)"(w3907) -> ()
          }
          frame #1 {
            n2373 = Wait (ms)(milliseconds to wait=w3920) -> ()  [unwired: 1 out]
          }
          frame #2 {
            n2374 = call "Write to pump.vi"("string"="start", "VISA resource name"=w3921) -> ()  [unwired: 1 out]
          }
        }
        n2375 = local read "Chemyx Syringe Pump Serial Port"() -> (w3903:refnum<visa-resource-name>)
      }
      event "Sample Channel\nFlow": Value Change {
        n2376 = event-data() -> ()  [unwired: 7 out]
        n2377 = Select(t="irun" ("string"), s="Sample Channel\nFlow", f="stop" ("string")) -> (s? t:f=w3925:string)
        n2378 = Concatenate Strings(w3925, "\r") -> (w3928:string)
        n2379 = VISA Write(VISA resource name=w3923, write buffer=w3928) -> ()  [unwired: 1 in, 3 out]
      }
      event "Start Flow": Value Change {
        n2380 = event-data() -> ()  [unwired: 7 out]
        n2381 = local write "Sample Channel\nFlow"(TRUE ("Sample Channel\nFlow")) -> ()
        n2382 = local write "Start Flow"(FALSE ("Start Flow")) -> ()
        n2383 = Concatenate Strings("irun" ("string"), "\r") -> (w3934:string)
        n2384 = VISA Write(VISA resource name=w3930, write buffer=w3934) -> ()  [unwired: 1 in, 3 out]
      }
      event "Stop Flow": Value Change {
        w3936 = FALSE ("Stop Flow")
        n2385 = event-data() -> ()  [unwired: 7 out]
        n2386 = local write "Stop Flow"(w3936) -> ()
        n2387 = local write "Sample Channel\nFlow"(w3936) -> ()
        n2388 = Concatenate Strings("stop" ("string"), "\r") -> (w3939:string)
        n2389 = VISA Write(VISA resource name=w3937, write buffer=w3939) -> ()  [unwired: 1 in, 3 out]
      }
      event "Flow rate (uL/h)": Value Change {
        n2390 = event-data() -> ()  [unwired: 7 out]
        n2391 = Number To Decimal String(number="Flow rate (uL/h)") -> (decimal integer string=w3946:string)  [unwired: 1 in]
        n2392 = Concatenate Strings("irate  " ("string"), w3946, " u/h" ("string"), "\r") -> (w3945:string)
        n2393 = VISA Write(VISA resource name=w3942, write buffer=w3945) -> ()  [unwired: 1 in, 3 out]
      }
      event "Flush Sample": Value Change {
        n2394 = event-data() -> ()  [unwired: 7 out]
        n2395 = flat-sequence {
          tunnel: w3951 -> [w3979]
          tunnel: [w3959] -> w3950
          tunnel: [w3953] -> w3948
          tunnel: w3950 -> [w3983]
          tunnel: [w3983] -> w3949
          tunnel: w3948 -> [w3982]
          tunnel: w3949 -> [w3988]
          frame #0 {
            # "set paramaters (rate, volume) for flush, clear volume"
            n2396 = Number To Decimal String(number="Flush rate (uL/m)") -> (decimal integer string=w3975:string)  [unwired: 1 in]
            n2397 = Concatenate Strings("irate  " ("string"), w3975, " u/m" ("string"), "\r") -> (w3977:string)
            n2398 = VISA Write(VISA resource name=w3979, write buffer=w3977) -> (VISA resource name out=w3973:refnum<visa-resource-name>)  [unwired: 1 in, 2 out]
            n2399 = Reciprocal(x="Flush rate (uL/m)") -> (1/x=w3956:dbl)
            n2400 = Number To Decimal String(number="Volume (uL)") -> (decimal integer string=w3964:string)  [unwired: 1 in]
            n2401 = Multiply(x="Volume (uL)", y=w3956) -> (x*y=w3955:dbl)
            n2402 = Concatenate Strings("tvolume  " ("string"), w3964, " u" ("string"), "\r") -> (w3962:string)
            n2403 = Multiply(x=w3955, y=60000.0) -> (x*y=w3953:dbl)
            n2404 = VISA Write(VISA resource name=w3973, write buffer=w3962) -> (VISA resource name out=w3961:refnum<visa-resource-name>)  [unwired: 1 in, 2 out]
            n2405 = Concatenate Strings("cvolume" ("string"), "\r") -> (w3960:string)
            n2406 = VISA Write(VISA resource name=w3961, write buffer=w3960) -> (VISA resource name out=w3971:refnum<visa-resource-name>)  [unwired: 1 in, 2 out]
            n2407 = Concatenate Strings("irun" ("string"), "\r") -> (w3969:string)
            n2408 = VISA Write(VISA resource name=w3971, write buffer=w3969) -> (VISA resource name out=w3959:refnum<visa-resource-name>)  [unwired: 1 in, 2 out]
          }
          frame #1 {
            # "Have to wait until\nflow is done to reset\nrate"
            n2409 = Add(x=w3982, y=100.0) -> (x+y=w3981:dbl)
            n2410 = Wait (ms)(milliseconds to wait=w3981) -> ()  [unwired: 1 out]
          }
          frame #2 {
            # "reset flow rate to usual flow rate"
            n2411 = local read "Flow rate (uL/h)"() -> (w3994:dbl)
            n2412 = Number To Decimal String(number=w3994) -> (decimal integer string=w3992:string)  [unwired: 1 in]
            n2413 = Concatenate Strings("irate  " ("string"), w3992, " u/h" ("string"), "\r") -> (w3990:string)
            n2414 = VISA Write(VISA resource name=w3988, write buffer=w3990) -> (VISA resource name out=w3984:refnum<visa-resource-name>)  [unwired: 1 in, 2 out]
            n2415 = Concatenate Strings("cvolume" ("string"), "\r") -> (w3985:string)
            n2416 = VISA Write(VISA resource name=w3984, write buffer=w3985) -> ()  [unwired: 1 in, 3 out]
          }
        }
      }
      event "Flush Pump 3": Value Change {
        n2417 = event-data() -> ()  [unwired: 7 out]
        n2418 = flat-sequence {
          tunnel: w3995 -> [w3998]
          frame #0 {
            # "set paramaters (rate, volume) for flush, clear volume"
            n2419 = Number To Decimal String(number="Flush rate (uL/m) P3") -> (decimal integer string=w4020:string)  [unwired: 1 in]
            n2420 = local write "Inject Pump 3"(TRUE ("Inject Pump 3")) -> ()
            n2421 = Concatenate Strings("irate  " ("string"), w4020, " u/m" ("string"), "\r") -> (w4022:string)
            n2422 = VISA Write(VISA resource name=w3998, write buffer=w4022) -> (VISA resource name out=w4018:refnum<visa-resource-name>)  [unwired: 1 in, 2 out]
            n2423 = Reciprocal(x="Flush rate (uL/m) P3") -> (1/x=w4002:dbl)
            n2424 = Number To Decimal String(number="Volume (uL) P3") -> (decimal integer string=w4009:string)  [unwired: 1 in]
            n2425 = Multiply(x="Volume (uL) P3", y=w4002) -> (x*y=w4001:dbl)
            n2426 = Concatenate Strings("tvolume  " ("string"), w4009, " u" ("string"), "\r") -> (w4007:string)
            n2427 = Multiply(x=w4001, y=60.0) -> (x*y=→"HP3 Flush Time (s)":dbl)
            n2428 = VISA Write(VISA resource name=w4018, write buffer=w4007) -> (VISA resource name out=w4006:refnum<visa-resource-name>)  [unwired: 1 in, 2 out]
            n2429 = Concatenate Strings("cvolume" ("string"), "\r") -> (w4005:string)
            n2430 = VISA Write(VISA resource name=w4006, write buffer=w4005) -> (VISA resource name out=w4016:refnum<visa-resource-name>)  [unwired: 1 in, 2 out]
            n2431 = Concatenate Strings("irun" ("string"), "\r") -> (w4014:string)
            n2432 = VISA Write(VISA resource name=w4016, write buffer=w4014) -> ()  [unwired: 1 in, 3 out]
          }
          frame #1 {
            "Flushing P3" <- TRUE ("Flushing P3")
          }
        }
      }
      event "Flush Pump 1": Value Change {
        n2433 = event-data() -> ()  [unwired: 7 out]
        n2434 = flat-sequence {
          tunnel: [w4036] -> w4026
          tunnel: w4025 -> [w4029]
          tunnel: w4026 -> [_]
          frame #0 {
            # "set paramaters (rate, volume) for flush, clear volume"
            n2435 = local write "Inject Pump 1"(TRUE ("Inject Pump 1")) -> ()
            n2436 = Number To Decimal String(number="Flush rate (uL/m) P1") -> (decimal integer string=w4052:string)  [unwired: 1 in]
            n2437 = Concatenate Strings("irate  " ("string"), w4052, " u/m" ("string"), "\r") -> (w4054:string)
            n2438 = VISA Write(VISA resource name=w4029, write buffer=w4054) -> (VISA resource name out=w4050:refnum<visa-resource-name>)  [unwired: 1 in, 2 out]
            n2439 = Reciprocal(x="Flush rate (uL/m) P1") -> (1/x=w4033:dbl)
            n2440 = Number To Decimal String(number="Volume (uL) P1") -> (decimal integer string=w4041:string)  [unwired: 1 in]
            n2441 = Multiply(x="Volume (uL) P1", y=w4033) -> (x*y=w4032:dbl)
            n2442 = Concatenate Strings("tvolume  " ("string"), w4041, " u" ("string"), "\r") -> (w4039:string)
            n2443 = Multiply(x=w4032, y=60.0) -> (x*y=→"HP1 Flush Time (s)":dbl)
            n2444 = VISA Write(VISA resource name=w4050, write buffer=w4039) -> (VISA resource name out=w4038:refnum<visa-resource-name>)  [unwired: 1 in, 2 out]
            n2445 = Concatenate Strings("cvolume" ("string"), "\r") -> (w4037:string)
            n2446 = VISA Write(VISA resource name=w4038, write buffer=w4037) -> (VISA resource name out=w4048:refnum<visa-resource-name>)  [unwired: 1 in, 2 out]
            n2447 = Concatenate Strings("irun" ("string"), "\r") -> (w4046:string)
            n2448 = VISA Write(VISA resource name=w4048, write buffer=w4046) -> (VISA resource name out=w4036:refnum<visa-resource-name>)  [unwired: 1 in, 2 out]
          }
          frame #1 {
            "Flushing P1" <- TRUE ("Flushing P3")
          }
        }
      }
      event "Clear Volume": Value Change {
        n2449 = event-data() -> ()  [unwired: 7 out]
        n2450 = Concatenate Strings("cvolume" ("string"), "\r") -> (w4058:string)
        n2451 = VISA Write(VISA resource name=w4057, write buffer=w4058) -> ()  [unwired: 1 in, 3 out]
      }
      event "Clear Volume P3": Value Change {
        n2452 = event-data() -> ()  [unwired: 7 out]
        n2453 = Concatenate Strings("cvolume" ("string"), "\r") -> (w4064:string)
        n2454 = VISA Write(VISA resource name=w4063, write buffer=w4064) -> ()  [unwired: 1 in, 3 out]
        n2455 = local write "Clear Volume P3"(FALSE ("Clear Volume P3")) -> ()
      }
      event "Clear Volume P1": Value Change {
        n2456 = event-data() -> ()  [unwired: 7 out]
        n2457 = Concatenate Strings("cvolume" ("string"), "\r") -> (w4069:string)
        n2458 = local write "Clear Volume P1"(FALSE ("Clear Volume P1")) -> ()
        n2459 = VISA Write(VISA resource name=w4068, write buffer=w4069) -> ()  [unwired: 1 in, 3 out]
      }
      event "Display On P3": Value Change {
        n2460 = event-data() -> ()  [unwired: 7 out]
        n2461 = Select(t="dim 100", s="Display On P3", f="dim 0") -> (s? t:f=w4075:string)
        n2462 = Concatenate Strings(w4075, "\r") -> (w4077:string)
        n2463 = VISA Write(VISA resource name=w4072, write buffer=w4077) -> ()  [unwired: 1 in, 3 out]
      }
      event "Display On P1": Value Change {
        n2464 = event-data() -> ()  [unwired: 7 out]
        n2465 = Select(t="dim 100", s="Display On P1", f="dim 0") -> (s? t:f=w4082:string)
        n2466 = Concatenate Strings(w4082, "\r") -> (w4084:string)
        n2467 = VISA Write(VISA resource name=w4079, write buffer=w4084) -> ()  [unwired: 1 in, 3 out]
      }
      event "Retract Pump 3": Value Change {
        n2468 = event-data() -> ()  [unwired: 7 out]
        n2469 = local write "Retract Pump 3"(FALSE ("Retract Pump 3")) -> ()
        n2470 = case shown="True" "Retract Pump 3" {
          tunnel: w4086 -> [_ w4089]
          frame False {
          }
          frame True {
            n2471 = Number To Decimal String(number="Retract Rate (uL/m)") -> (decimal integer string=w4107:string)  [unwired: 1 in]
            n2472 = Concatenate Strings("wrate  " ("string"), w4107, " u/m" ("string"), "\r") -> (w4109:string)
            n2473 = VISA Write(VISA resource name=w4089, write buffer=w4109) -> (VISA resource name out=w4100:refnum<visa-resource-name>)  [unwired: 1 in, 2 out]
            n2474 = Number To Decimal String(number="Retract Vol 3 (uL)") -> (decimal integer string=w4102:string)  [unwired: 1 in]
            n2475 = Concatenate Strings("tvolume  " ("string"), w4102, " u" ("string"), "\r") -> (w4099:string)
            n2476 = VISA Write(VISA resource name=w4100, write buffer=w4099) -> (VISA resource name out=w4095:refnum<visa-resource-name>)  [unwired: 1 in, 2 out]
            n2477 = Concatenate Strings("cvolume" ("string"), "\r") -> (w4096:string)
            n2478 = VISA Write(VISA resource name=w4095, write buffer=w4096) -> (VISA resource name out=w4090:refnum<visa-resource-name>)  [unwired: 1 in, 2 out]
            n2479 = Concatenate Strings("wrun" ("string"), "\r") -> (w4091:string)
            n2480 = VISA Write(VISA resource name=w4090, write buffer=w4091) -> ()  [unwired: 1 in, 3 out]
          }
        }
      }
      event "Retract Pump 1": Value Change {
        n2481 = event-data() -> ()  [unwired: 7 out]
        n2482 = local write "Retract Pump 1"(FALSE ("Retract Pump 1")) -> ()
        n2483 = case shown="True" "Retract Pump 1" {
          tunnel: w4111 -> [_ w4116]
          frame False {
          }
          frame True {
            n2484 = local read "Retract Rate (uL/m)"() -> (w4114:dbl)
            n2485 = Number To Decimal String(number=w4114) -> (decimal integer string=w4132:string)  [unwired: 1 in]
            n2486 = Concatenate Strings("wrate  " ("string"), w4132, " u/m" ("string"), "\r") -> (w4134:string)
            n2487 = VISA Write(VISA resource name=w4116, write buffer=w4134) -> (VISA resource name out=w4126:refnum<visa-resource-name>)  [unwired: 1 in, 2 out]
            n2488 = Number To Decimal String(number="Retract Vol 1 (uL)") -> (decimal integer string=w4128:string)  [unwired: 1 in]
            n2489 = Concatenate Strings("tvolume  " ("string"), w4128, " u" ("string"), "\r") -> (w4125:string)
            n2490 = VISA Write(VISA resource name=w4126, write buffer=w4125) -> (VISA resource name out=w4122:refnum<visa-resource-name>)  [unwired: 1 in, 2 out]
            n2491 = Concatenate Strings("cvolume" ("string"), "\r") -> (w4123:string)
            n2492 = VISA Write(VISA resource name=w4122, write buffer=w4123) -> (VISA resource name out=w4117:refnum<visa-resource-name>)  [unwired: 1 in, 2 out]
            n2493 = Concatenate Strings("wrun" ("string"), "\r") -> (w4118:string)
            n2494 = VISA Write(VISA resource name=w4117, write buffer=w4118) -> ()  [unwired: 1 in, 3 out]
          }
        }
      }
      event "Flip Green Filter": Value Change {
        n2495 = event-data() -> ()  [unwired: 7 out]
        n2496 = Not(x="Flip Green Filter") -> (.not. x?=w4136:bool)
        n2497 = local write "Flip Green Filter"(w4136) -> ()
        n2498 = flat-sequence {
          tunnel: w4144 -> [w4149]
          tunnel: w4143 -> [w4148]
          tunnel: [w4146] -> w4141
          tunnel: [w4145] -> w4140
          tunnel: [w4151] -> w4139
          tunnel: w4141 -> [w4151]
          tunnel: [w4150] -> w4138
          tunnel: w4140 -> [w4150]
          tunnel: w4139 -> [w4155]
          tunnel: w4138 -> [w4154]
          tunnel: [w4153] -> w4142
          frame #0 {
            n2499 = xnode "Read/Write Control"("FPGA VI Reference In"=w4149, "error in"=w4148, "Green Filter Flipper"=TRUE) -> ("FPGA VI Reference Out"=w4146:T18, "error out"=w4145:errorcluster)
          }
          frame #1 {
            n2500 = Wait (ms)(milliseconds to wait=u32 100) -> ()  [unwired: 1 out]
          }
          frame #2 {
